vi "GetAllData.vi"(8 "error In":errorcluster, 11 "VISA resource In":refnum<visa-resource-name>) -> (0 "error out":errorcluster, 2 "Data Out":u16[](array[numeric]), 3 "VISA resource Out":refnum<visa-resource-name>)   [LabVIEW 2009]
uses:
  Packet.ctl
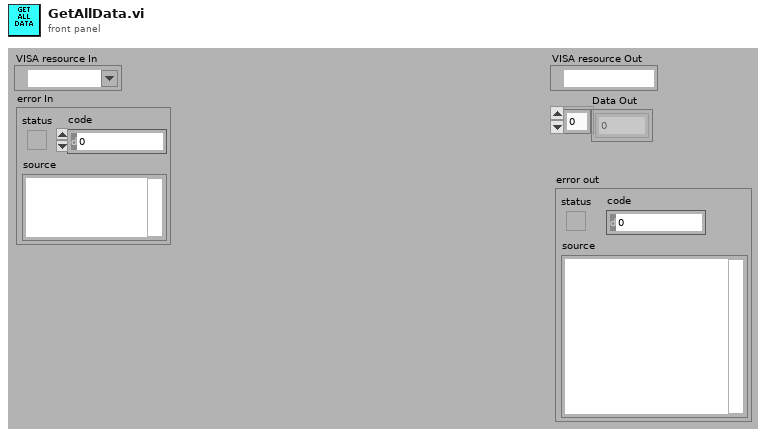
[diagram p1: front panel]
types:
  T1 = typedef "Packet.ctl" = cluster{"Length":u8, "Type":u8, "PID":u8, "Data":u8[], "CRC":u8}
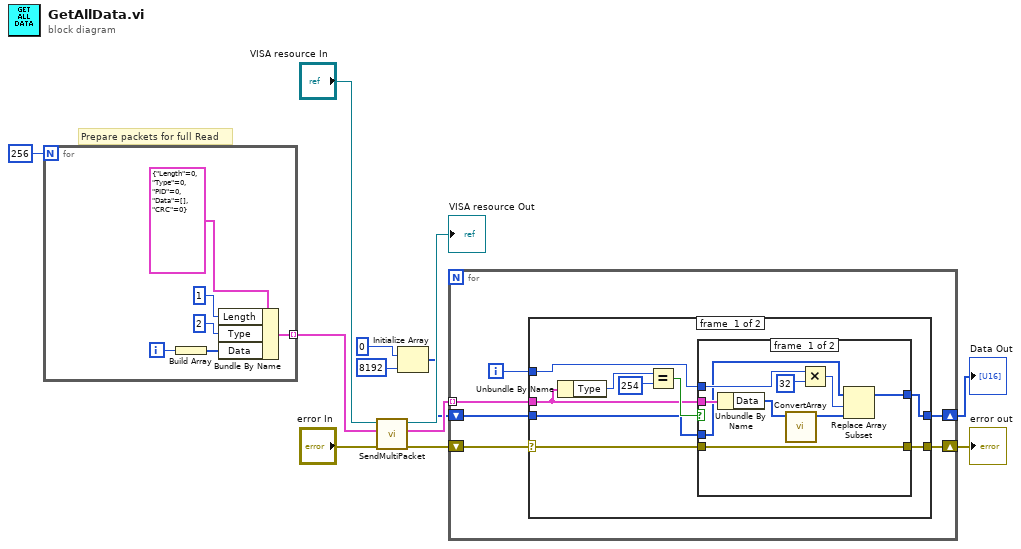
[diagram p0: block diagram]
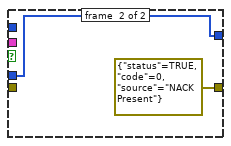
[diagram p2: hidden frame]
diagram:
  # "Prepare packets for full Read"
  n1 = for {
    N: 256 -> [_]
    tunnel: [w13] -> w6 mode=indexing
    i -> [w15]
    n2 = Build Array(w15) -> (w14:i32[])
    n3 = Bundle By Name(cluster=T1 {"Length"=0, "Type"=0, "PID"=0, "Data"=[], "CRC"=0} ("Transmit"), "Length"=u8 1, "Type"=u8 2, "Data"=w14) -> (w13:T1)
  }
  n4 = call "SendMultiPacket.vi"("error in (no error)"="error In", "Packets In"=w6, "VISA resource name"="VISA resource In") -> ("error out"=w2:errorcluster, "ReceivedBytes"=w3:T1[], "VISA resource name out"=→"VISA resource Out":refnum<visa-resource-name>)  [unwired: 5 in, 1 out]
  n5 = Initialize Array(u16 0, 8192 ("dimension size")) -> (w1:u16[])
  n6 = for {
    shift-right: [w23] -> w10
    shift-left: w1 -> [w20]
    shift-right: [w24] -> w11
    shift-left: w2 -> [w21]
    tunnel: w3 -> [w22] mode=indexing
    i -> [w19]
    n7 = case shown="No Error" w21 {
      selector: w21 -> [w27 w46]
      tunnel: [w30 w46] -> w24
      tunnel: [w29 w45] -> w23
      tunnel: w22 -> [w28 _]
      tunnel: w20 -> [w26 w45]
      tunnel: w19 -> [w25 _]
      frame #0 {
        n8 = Unbundle By Name(w28) -> ("Type"=w31:u8)
        n9 = Equal?(x=w31, y=u8 254) -> (x = y?=w33:bool)
        n10 = case shown="True" w33 {
          tunnel: w27 -> [w42 _]
          tunnel: [w42 errorcluster {"status"=TRUE, "code"=0, "source"="NACK Present"} ("error IO")] -> w30
          tunnel: w28 -> [w41 _]
          tunnel: w26 -> [w34 w43]
          tunnel: [w40 w43] -> w29
          tunnel: w25 -> [w39 _]
          frame #0 {
            n11 = Unbundle By Name(w41) -> ("Data"=w36:u8[])
            n12 = call "ConvertArray.vi"("Data In"=w36) -> ("Data Out"=w35:u16[])  [unwired: 10 in]
            n13 = Multiply(x=w39, y=32) -> (x*y=w37:i32)
            n14 = Replace Array Subset(array=w34, new element=w35, index=w37) -> (w40:u16[])
          }
          frame #1 {
          }
        }
      }
      frame #1 {
      }
    }
  }
  "error out" <- w11
  "Data Out" <- w10
